vi "OpenProcessOnError.vi"(1 "Open?":bool, 5 "Error In":errorcluster) -> (19 "Error Out":errorcluster)   [LabVIEW 2019, in "Error handler.lvclass"]
uses:
  Error handler.lvclass
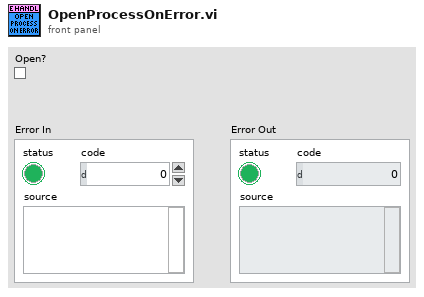
[diagram p1: front panel]
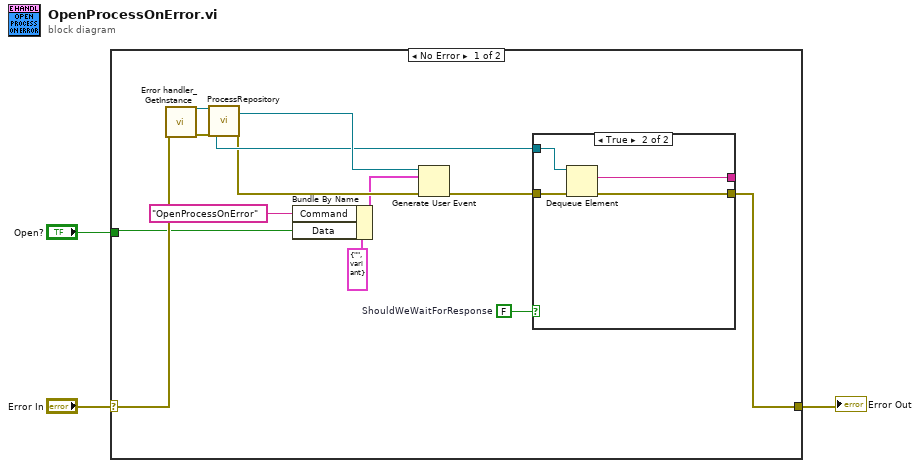
[diagram p0: block diagram]
diagram:
  n1 = case shown="No Error" "Error In" {
    selector: "Error In" -> [w7 w22]
    tunnel: [w6 w22] -> w2
    tunnel: "Open?" -> [w5 _]
    frame No Error {
      w15 = FALSE  # ShouldWeWaitForResponse
      n2 = call "Error handler_GetInstance.vi"("error in"=w7) -> ("reference out"=w11:refnum<class "Error handler.lvclass">, "error out"=w10:errorcluster)  [unwired: 14 in, 3 out]
      n3 = call "ProcessRepository.vi"("reference in"=w11, "Error In"=w10) -> ("QueueFromProcess"=w13:refnum<queue>, "EventsToProcess"=w16:refnum<user-event>, "Error Out"=w12:errorcluster)  [unwired: 10 in, 5 out]
      n4 = Bundle By Name(cluster=cluster{"Command":string, "Data":variant} {"Command"="", "Data"=variant} ("MessageToProcess"), "Command"="OpenProcessOnError", "Data"=w5) -> (w8:cluster{"Command":string, "Data":variant})
      n5 = Generate User Event(user event=w16, event data cluster=w8, error in=w12) -> (error out=w14:errorcluster)  [unwired: 1 in, 1 out]
      n6 = case shown="True" w15 {
        tunnel: w14 -> [w17 w21]
        tunnel: w13 -> [_ w20]
        tunnel: [_ w19] -> _
        tunnel: [w17 w18] -> w6
        frame False {
        }
        frame True {
          n7 = Dequeue Element(queue=w20, error in (no error)=w21) -> (element=w19:string, error out=w18:errorcluster)  [unwired: 1 in, 2 out]
        }
      }
    }
    frame Error {
    }
  }
  "Error Out" <- w2
